vi "solar_excel Import.vi"(6 "Visible? (F)":bool, 8 "error in (no error)":errorcluster, 10 "Excel Workbook (*.xlsx)":path, 11 "TSV Workbook (*.tsv)":path) -> (0 "error out":errorcluster, 3 "Excel Workbook out":path)   [LabVIEW 2018]
doc: "This imports a tab delimited text file (*.tsv) to an Excel Workbook (*.xlsx). The sections in the tab delimited text file specify the corresponding Worksheet.\n\n[MySheet1] <- Creates a 'MySheet1' worksheet\nA\\tB\\tC\nD\\tE\\tF"
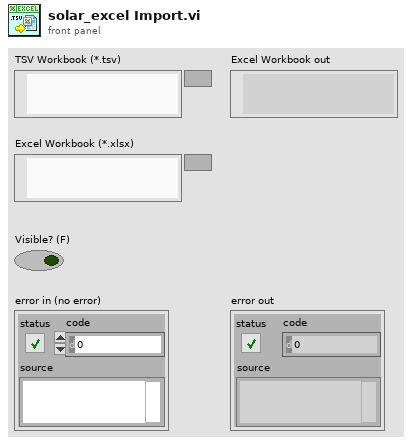
[diagram p1: front panel]
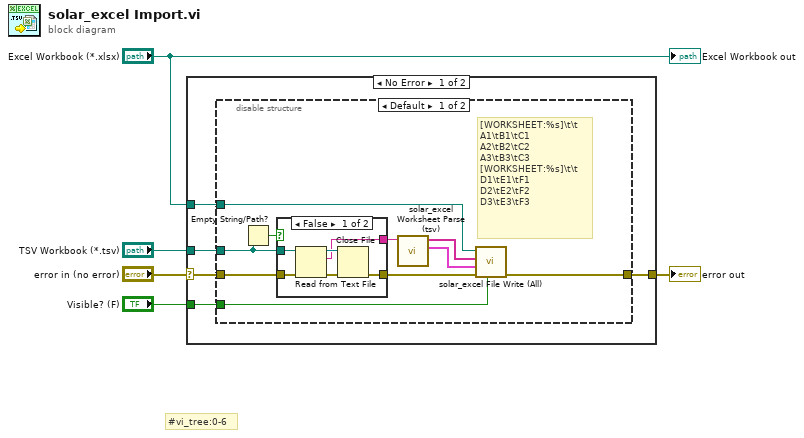
[diagram p0: block diagram]
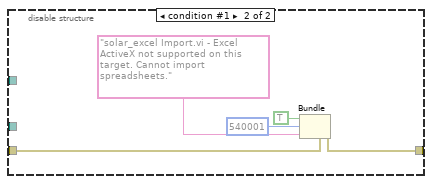
[diagram p3: hidden frame]
diagram:
  # "#vi_tree:0-6"
  n1 = case shown="No Error" "error in (no error)" {
    selector: "error in (no error)" -> [w9 w33]
    tunnel: [w8 w33] -> w4
    tunnel: "Excel Workbook (*.xlsx)" -> [w6 _]
    tunnel: "Visible? (F)" -> [w7 _]
    tunnel: "TSV Workbook (*.tsv)" -> [w10 _]
    frame No Error {
      n2 = disable-structure shown="Default" {
        disable-tunnel: w10 -> [w20 _]
        disable-tunnel: w9 -> [w18 w30]
        disable-tunnel: [w15 w29] -> w8
        disable-tunnel: w7 -> [w14 _]
        disable-tunnel: w6 -> [w11 _]
        frame condition #0 (active) {
          # "[WORKSHEET:%s]\\t\\t\nA1\\tB1\\tC1\nA2\\tB2\\tC2\nA3\\tB3\\tC3\n[WORKSHEET:%s]\\t\\t\nD1\\tE1\\tF1\nD2\\tE2\\tF2\nD3\\tE3\\tF3"
          n3 = Empty String/Path?(string/path=w20) -> (empty?=w19:bool)
          n4 = case shown="False" w19 {
            tunnel: w20 -> [w25 _]
            tunnel: [w26 w27] -> w16
            tunnel: [w22 _] -> w17
            tunnel: w18 -> [w21 w27]
            frame False {
              n5 = Read from Text File(file (use dialog)=w25, error in=w21) -> (refnum out=w23:refnum<file>, text=w22:string, error out=w24:errorcluster)  [unwired: 2 in, 1 out]
              n6 = Close File(refnum=w23, error in=w24) -> (error out=w26:errorcluster)  [unwired: 1 out]
            }
            frame True {
            }
          }
          n7 = call "solar_excel Worksheet Parse (tsv).vi"("Tab Delimited String"=w17) -> ("Worksheets Cells"=w13:cluster{"Cells":string[][]}[], "Worksheets"=w12:string[])  [unwired: 9 in]
          n8 = call "solar_excel File Write (All).vi"("Visible? (F)"=w14, "error in (no error)"=w16, "Worksheets Cells"=w13, "Worksheets"=w12, "Excel Workbook (*.xlsx)"=w11) -> ("error out"=w15:errorcluster)  [unwired: 5 in, 1 out]
        }
        frame condition #1 {
          n9 = Bundle(cluster=w30, "status"=TRUE ("show call chain? (False)"), "code"=540001 ("error code (0)"), "source"="solar_excel Import.vi - Excel ActiveX not supported on this target. Cannot import spreadsheets." ("error message (\"\")")) -> (w29:errorcluster)
        }
      }
    }
    frame Error {
    }
  }
  "error out" <- w4
  "Excel Workbook out" <- "Excel Workbook (*.xlsx)"
